vi "Configure Math Expression.vi"(5 "Math Expression Unit (W)":string="W", 6 "Enable Math Expression (F: Disable)":bool, 7 "Expression Definition (VOLT*CURR)":string="(VOLT*CURR)", 8 "error in (no error)":errorcluster, 9 "Expression Name (MyMath1)":string="MyMath1", 10 "Channel (0: Channel 1)":i32(ring) items=["Channel 1", "Channel 2"], 11 "VISA resource name":refnum<visa-resource-name>) -> (0 "error out":errorcluster, 3 "VISA resource name out":refnum<visa-resource-name>)   [LabVIEW 2020, in "Agilent B2900 Series.lvlib"]
doc: "Defines a math expression to perform the Limit Test Calculation ."
uses:
  Agilent B2900 Series.lvlib
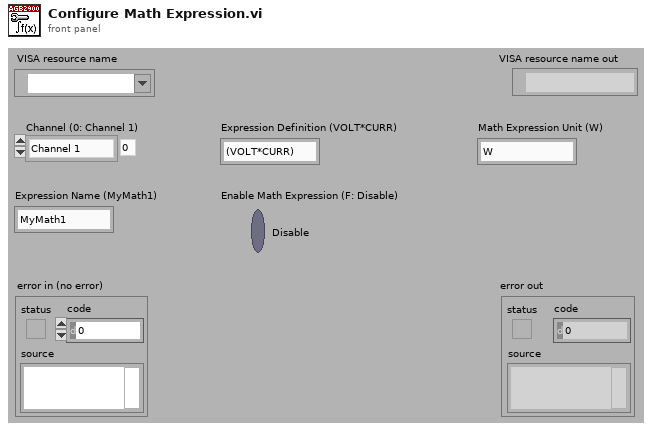
[diagram p1: front panel]
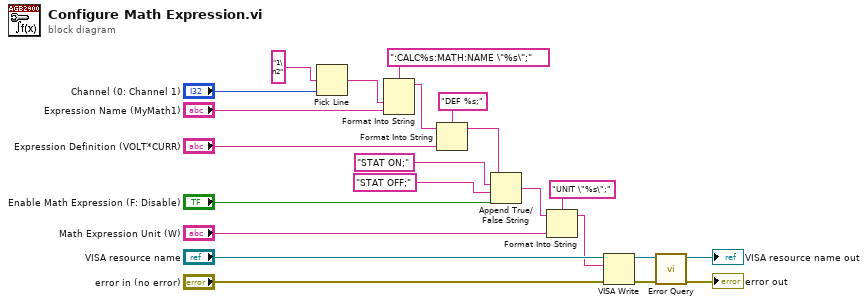
[diagram p0: block diagram]
diagram:
  n1 = Pick Line(multi-line string="1\n2" ("string (\"\")"), line index="Channel (0: Channel 1)") -> (output string=w5:string)  [unwired: 1 in]
  n2 = Format Into String(format string=":CALC%s:MATH:NAME \"%s\";", w5, "Expression Name (MyMath1)") -> (resulting string=w20:string)  [unwired: 2 in, 1 out]
  n3 = Format Into String(format string="DEF %s;", initial string=w20, "Expression Definition (VOLT*CURR)") -> (resulting string=w2:string)  [unwired: 1 in, 1 out]
  n4 = Append True/False String(1:"Enable Math Expression (F: Disable)", 2:"STAT OFF;", 3:"STAT ON;", 4:w2) -> (0:w14:string)
  n5 = Format Into String(format string="UNIT \"%s\";", initial string=w14, "Math Expression Unit (W)") -> (resulting string=w1:string)  [unwired: 1 in, 1 out]
  n6 = VISA Write(VISA resource name="VISA resource name", write buffer=w1, error in (no error)="error in (no error)") -> (VISA resource name out=w9:refnum<visa-resource-name>, error out=w8:errorcluster)  [unwired: 1 out]
  n7 = call "Error Query.vi"("error in (no error)"=w8, "VISA resource name"=w9) -> ("error out"=→"error out":errorcluster, "VISA resource name out"=→"VISA resource name out":refnum<visa-resource-name>)  [unwired: 6 in, 2 out]
